vi "Read Attributes.vi"(5 "Flatten Pointer?":bool, 7 "Linked List ID":string, 8 "error in (no error)":errorcluster, 10 "Include Private?":bool, 11 "Linked List Ref":refnum<data-value>) -> (0 "error out":errorcluster, 1 "Attributes":variant[](array[variant]), 2 "Attribute Names out":string[](array[string]), 3 "Linked List Ref out":refnum<data-value>, 4 "found":bool, 6 "Data IDs":string[](array[string]))   [LabVIEW 2020, in "Linked Lists.lvlib" / "Linked List Ref.lvclass"]
uses:
  <vilib>/gpm_packages/@cs/linked-list/Source/Linked List/Linked List Ref/Linked List Ref.lvclass
  <vilib>/gpm_packages/@cs/linked-list/Source/Linked List/ILinkedList/ILinked List.lvclass
panel:
  out "Missing GUIDs out":string[](array[string])
  in  "Attribute Names":string[](array[string])
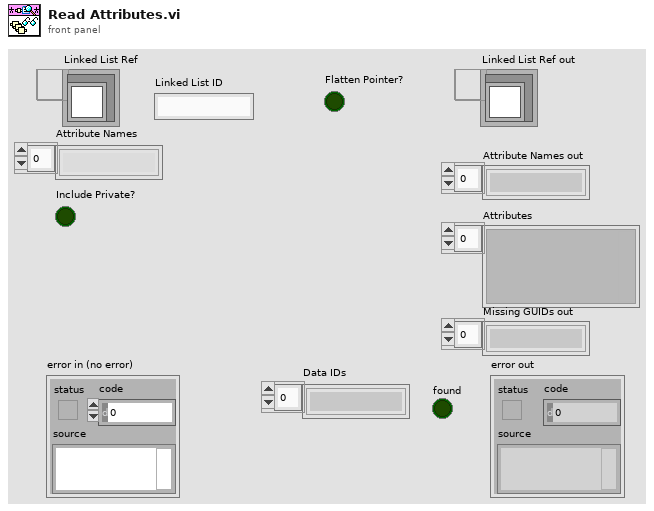
[diagram p1: front panel]
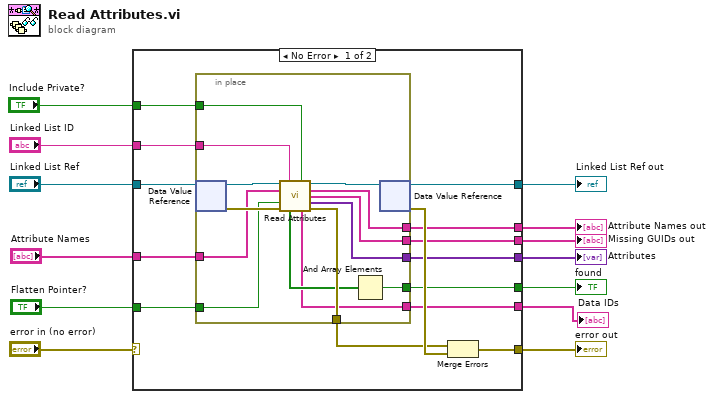
[diagram p0: block diagram]
diagram:
  n1 = case shown="No Error" "error in (no error)" {
    selector: "error in (no error)" -> [_ w43]
    tunnel: "Linked List Ref" -> [w27 w42]
    tunnel: "Linked List ID" -> [w26 _]
    tunnel: [w24 w43] -> w10
    tunnel: [w25 w42] -> w9
    tunnel: [w21 _] -> w8
    tunnel: "Attribute Names" -> [w20 _]
    tunnel: [w19 _] -> w5
    tunnel: [w18 _] -> w6
    tunnel: "Flatten Pointer?" -> [w17 _]
    tunnel: [w16 _] -> w3
    tunnel: "Include Private?" -> [w15 _]
    tunnel: [w14 _] -> w1
    frame No Error {
      n2 = in-place {
        in-place-border: w26 -> [w37]
        in-place-border: [w38] -> w22
        in-place-border: [w34] -> w21
        in-place-border: w20 -> [w36]
        in-place-border: [w33] -> w19
        in-place-border: [w32] -> w18
        in-place-border: w17 -> [w31]
        in-place-border: [w30] -> w16
        in-place-border: w15 -> [w29]
        in-place-border: [w28] -> w14
        n3 = in-place-dvr #1(w27) -> (w41:refnum<class "ILinked List.lvclass">, w39:errorcluster)
        n4 = call-dynamic "Read Attributes.vi"("ILinked List in"=w41, "Linked List ID"=w37, "Include Private?"=w29, "Attribute Names"=w36, "Flatten Pointer?"=w31, "error in (no error)"=w39) -> ("ILinked List out"=w40:refnum<class "ILinked List.lvclass">, "Attribute Names out"=w32:string[], "Missing GUIDs out"=w28:string[], "Attributes"=w33:variant[], "Found?"=w35:bool[], "Data IDs"=w30:string[], "error out"=w38:errorcluster)  [unwired: 3 in]
        n5 = And Array Elements(Boolean array=w35) -> (logical AND=w34:bool)
        n6 = in-place-dvr #1(w40) -> (w25:refnum<data-value>, w23:errorcluster)
      }
      n7 = Merge Errors(w22, w23) -> (w24:errorcluster)
    }
    frame Error {
    }
  }
  "error out" <- w10
  "Linked List Ref out" <- w9
  "found" <- w8
  "Attribute Names out" <- w6
  "Attributes" <- w5
  "Data IDs" <- w3
  "Missing GUIDs out" <- w1
